vi "EnableDisableControlls.vi"(8 "error in (no error)":errorcluster, 10 "State":T1, 11 "Common Refs":T2={"LBox_ChList"=refnum, "OXY_SCPI Ref"="TCPIP0::192.168.1.75::10001::SOCKET", "STR_ChName1"=refnum, "STR_ChName2"=refnum, "STR_ChName3"=refnum, "STR_ChName4"=refnum, "STR_ChName5"=refnum, "STR_ChName6"=refnum, "Button_Stop"=refnum, "Button_Start"=refnum, "Button_Disconnect"=refnum, "Button_Connect"=refnum, "Bool_StatusLED"=refnum, "DS Ref"="TCPIP0::192.168.1.75::10001::SOCKET", "Button_SetPort"=refnum, "Button_GetPort"=refnum, "Button_GetState"=refnum, "Button_Reset"=refnum, "Button_Init"=refnum, "STR_UserCMD"=refnum, "STR_CmdPromp"=refnum, "Port"=refnum, "Button_QuerryChs"=refnum, "Graph"=refnum, "STR_ConnAddress"=refnum}) -> (0 "error out":errorcluster)   [LabVIEW 2020]
uses:
  TypeDefs/Refs_Common.ctl
  <vilib>/Stadlmann TEC/OXYGEN Datastream/VIs/Setup/TypeDefs/States.ctl
  <vilib>/Stadlmann TEC/OXYGEN Datastream/OXYGEN_Datastream.lvlib
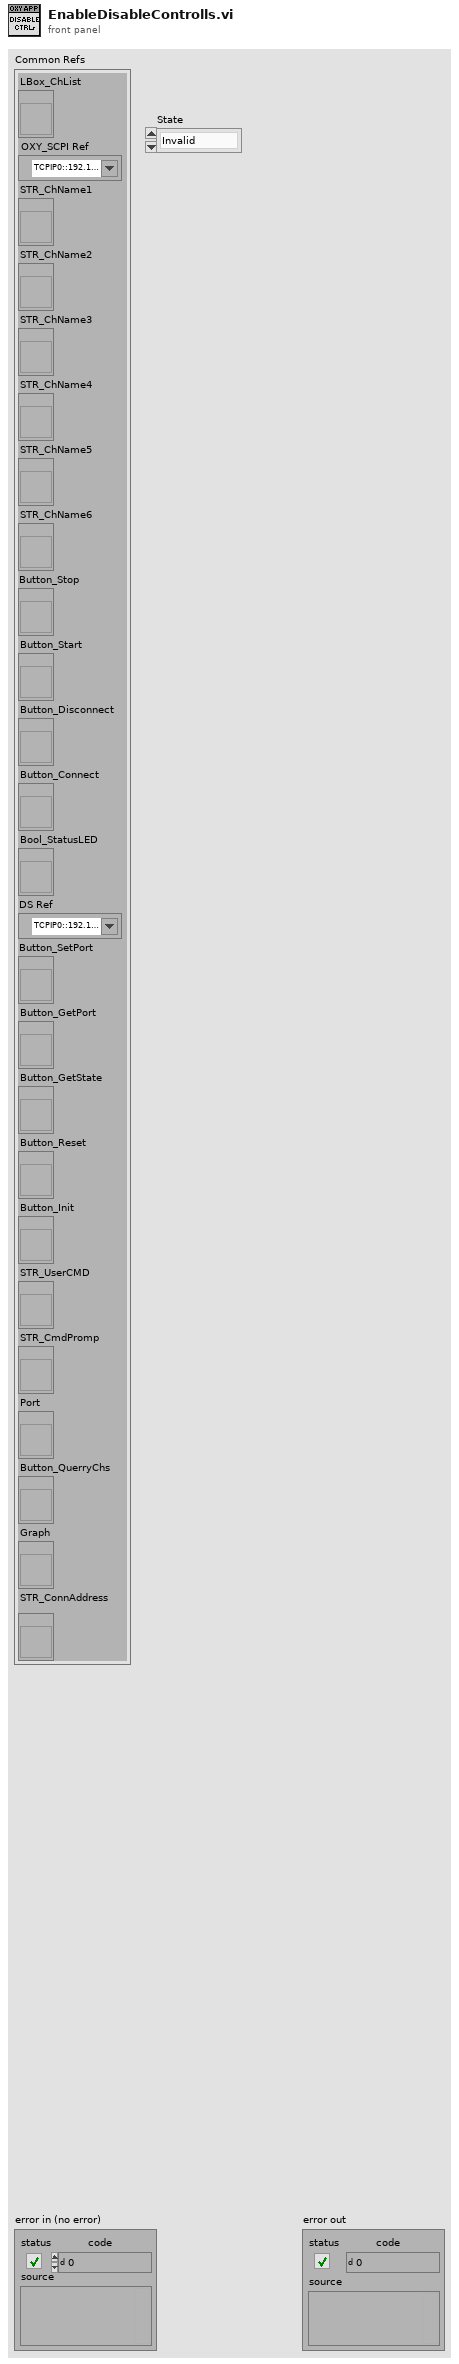
[diagram p1: front panel]
types:
  T1 = typedef "OXYGEN_Datastream.lvlib/States.ctl" = enum16{"Invalid", "Config", "Initialized", "Running", "Error", "Unlicensed"}
  T2 = typedef "Refs_Common.ctl" = cluster{"LBox_ChList":refnum<vi>, "OXY_SCPI Ref":refnum<visa-resource-name>, "STR_ChName1":refnum<vi>, "STR_ChName2":refnum<vi>, "STR_ChName3":refnum<vi>, "STR_ChName4":refnum<vi>, "STR_ChName5":refnum<vi>, "STR_ChName6":refnum<vi>, "Button_Stop":refnum<vi>, "Button_Start":refnum<vi>, "Button_Disconnect":refnum<vi>, "Button_Connect":refnum<vi>, "Bool_StatusLED":refnum<vi>, "DS Ref":refnum<visa-resource-name>, "Button_SetPort":refnum<vi>, "Button_GetPort":refnum<vi>, "Button_GetState":refnum<vi>, "Button_Reset":refnum<vi>, "Button_Init":refnum<vi>, "STR_UserCMD":refnum<vi>, "STR_CmdPromp":refnum<vi>, "Port":refnum<vi>, "Button_QuerryChs":refnum<vi>, "Graph":refnum<vi>, "STR_ConnAddress":refnum<vi>}
  T3 = enum8{"Enabled", "Disabled", "Disabled and Grayed Out"}
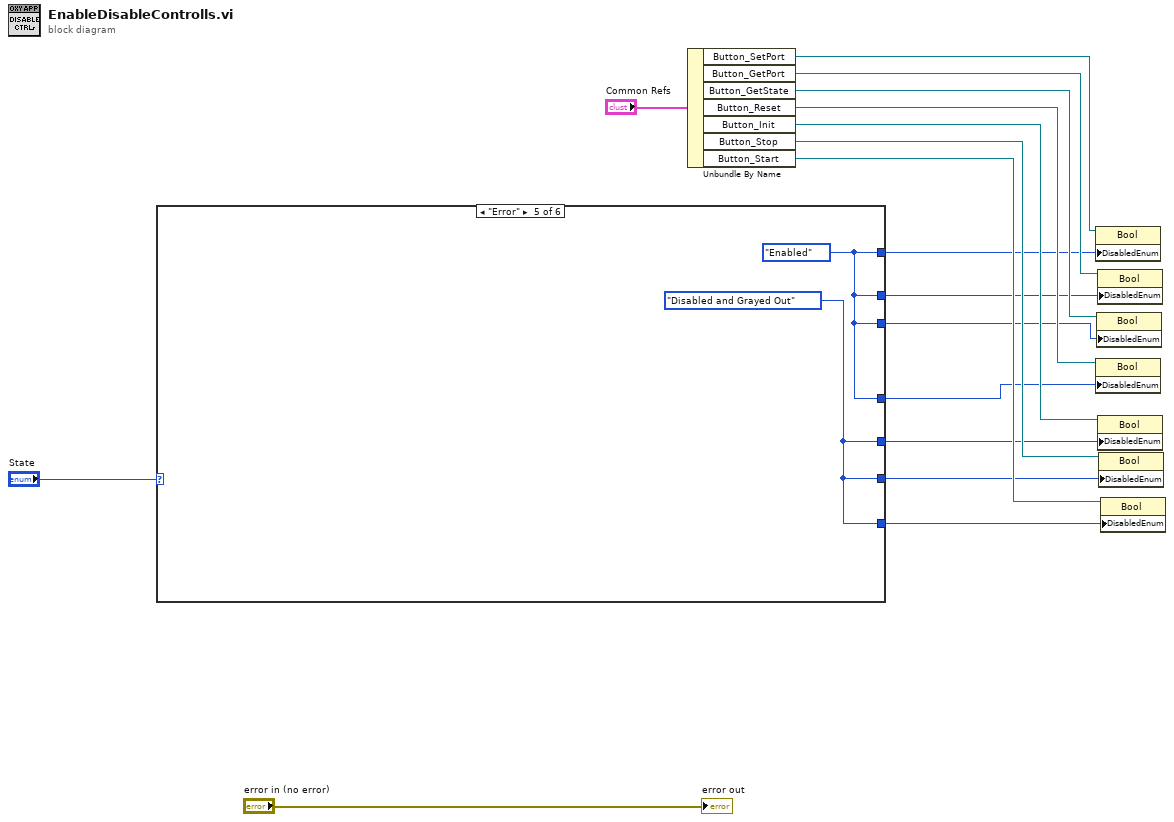
[diagram p0: block diagram]
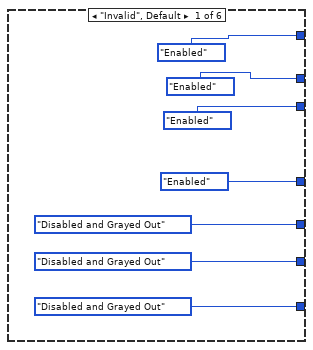
[diagram p2: hidden frame]
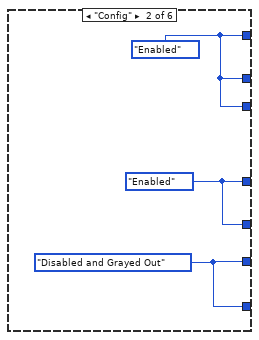
[diagram p3: hidden frame]
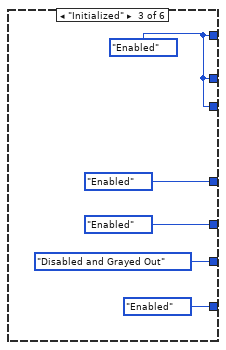
[diagram p4: hidden frame]
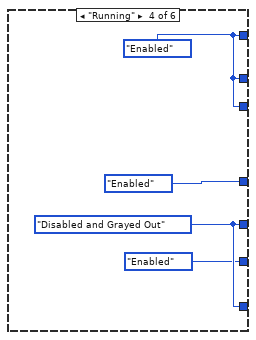
[diagram p5: hidden frame]
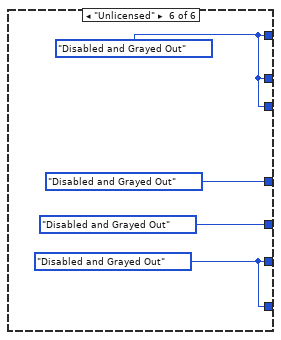
[diagram p6: hidden frame]
diagram:
  n1 = case shown="\"Error\"" "State" {
    tunnel: [T3."Enabled" ("Disabled") w27 T3."Enabled" ("Disabled") T3."Enabled" ("Disabled") w37 T3."Disabled and Grayed Out" ("Disabled")] -> w8
    tunnel: [T3."Disabled and Grayed Out" ("Disabled") w27 T3."Enabled" ("Disabled") w35 w38 T3."Disabled and Grayed Out" ("Disabled")] -> w7
    tunnel: [T3."Disabled and Grayed Out" ("Disabled") w26 T3."Disabled and Grayed Out" ("Disabled") T3."Enabled" ("Disabled") w38 w40] -> w6
    tunnel: [T3."Disabled and Grayed Out" ("Disabled") w26 T3."Enabled" ("Disabled") w35 w38 w40] -> w5
    tunnel: [T3."Enabled" ("Disabled") w25 w30 w33 w37 w39] -> w4
    tunnel: [T3."Enabled" ("Disabled") w25 w30 w33 w37 w39] -> w2
    tunnel: [T3."Enabled" ("Disabled") w25 w30 w33 w37 w39] -> w1
    frame "Invalid", Default {
    }
    frame "Config" {
      w25 = T3."Enabled" ("Disabled")
      w26 = T3."Disabled and Grayed Out" ("Disabled")
      w27 = T3."Enabled" ("Disabled")
    }
    frame "Initialized" {
      w30 = T3."Enabled" ("Disabled")
    }
    frame "Running" {
      w33 = T3."Enabled" ("Disabled")
      w35 = T3."Disabled and Grayed Out" ("Disabled")
    }
    frame "Error" {
      w38 = T3."Disabled and Grayed Out" ("Disabled")
      w37 = T3."Enabled" ("Disabled")
    }
    frame "Unlicensed" {
      w40 = T3."Disabled and Grayed Out" ("Disabled")
      w39 = T3."Disabled and Grayed Out" ("Disabled")
    }
  }
  n2 = Unbundle By Name("Common Refs") -> ("Button_SetPort"=w9:refnum<vi>, "Button_GetPort"=w10:refnum<vi>, "Button_GetState"=w11:refnum<vi>, "Button_Reset"=w12:refnum<vi>, "Button_Init"=w13:refnum<vi>, "Button_Stop"=w14:refnum<vi>, "Button_Start"=w15:refnum<vi>)
  n3 = property class="Bool"(reference=w9, "DisabledEnum"=w4) -> ()  [unwired: 1 in, 2 out]
  n4 = property class="Bool"(reference=w12, "DisabledEnum"=w8) -> ()  [unwired: 1 in, 2 out]
  n5 = property class="Bool"(reference=w11, "DisabledEnum"=w1) -> ()  [unwired: 1 in, 2 out]
  n6 = property class="Bool"(reference=w10, "DisabledEnum"=w2) -> ()  [unwired: 1 in, 2 out]
  n7 = property class="Bool"(reference=w13, "DisabledEnum"=w7) -> ()  [unwired: 1 in, 2 out]
  n8 = property class="Bool"(reference=w14, "DisabledEnum"=w6) -> ()  [unwired: 1 in, 2 out]
  n9 = property class="Bool"(reference=w15, "DisabledEnum"=w5) -> ()  [unwired: 1 in, 2 out]
  "error out" <- "error in (no error)"
